vi "PCSLauncher.ProcPeriodic.vi"(0 "i ref in":refnum<vi>, 3 "ms timeout (100)":i32=100, 5 "error in (no error)":errorcluster) -> (14 "i ref out":refnum<vi>, 17 "timed out":bool, 19 "error out":errorcluster)   [LabVIEW 2014, in "PCSLauncher.lvlib"]
doc: "This method serves to periodically do things like reading values from the HW. Methods that should be executed periodically should be called from THIS methode. Add code here."
uses:
  PCSLauncher.lvlib
  CS_Core/CSObj/CSObj.lvlib
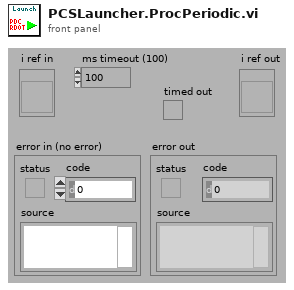
[diagram p1: front panel]
types:
  T1 = enum8{"Enabled", "Disabled", "Disabled and Grayed Out"}
  T2 = typedef "PCSLauncher.lvlib/PCSLauncher.i attribute.ctl" = cluster{"PCS Systems":cluster{"GUI Ref":refnum<vi>, "Super alive?":bool, "Start-GOG alive?":bool}[], "GUI Refs":cluster{"Delete":refnum<vi>, "Launch PCS":refnum<vi>}}
  T3 = cluster{"GUI Ref":refnum<vi>, "Super alive?":bool, "Start-GOG alive?":bool}[]
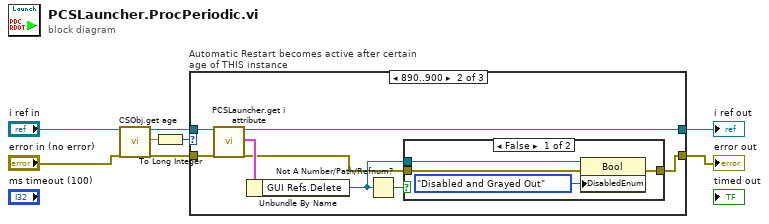
[diagram p0: block diagram]
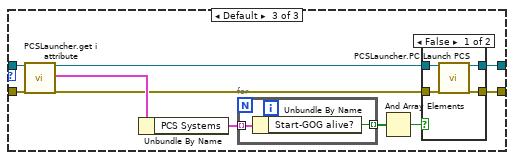
[diagram p4: hidden frame]
diagram:
  n1 = call "CSObj.get age.vi"("i ref in"="i ref in", "error in (no error)"="error in (no error)") -> ("i ref out"=w5:refnum<vi>, "age"=w1:dbl, "error out"=w3:errorcluster)  [unwired: 15 in]
  n2 = To Long Integer(number=w1) -> (32bit integer=w2:i32)
  n3 = case "Automatic Restart becomes active after certain age of THIS instance" shown="890..900" w2 {
    tunnel: [w10 w17 w30] -> w8
    tunnel: [w9 w11 w28] -> w7
    tunnel: w5 -> [w10 w18 w25]
    tunnel: w3 -> [w9 w16 w24]
    frame 0..889 {
    }
    frame 890..900 {
      n4 = call "PCSLauncher.get i attribute.vi"("i ref in"=w18, "error in (no error)"=w16) -> ("i ref out"=w17:refnum<vi>, "i attribute"=w15:T2, "error out"=w12:errorcluster)  [unwired: 15 in]
      n5 = Unbundle By Name(w15) -> ("GUI Refs.Delete"=w14:refnum<vi>)
      n6 = Not A Number/Path/Refnum?(number/path/refnum=w14) -> (NaN/Path/Refnum?=w13:bool)
      n7 = case shown="False" w13 {
        tunnel: w12 -> [w22 w23]
        tunnel: [w21 w23] -> w11
        tunnel: w14 -> [w20 _]
        frame False {
          n8 = property class="Bool"(reference=w20, error in=w22, "DisabledEnum"=T1."Disabled and Grayed Out" ("Disabled")) -> (error out=w21:errorcluster)  [unwired: 1 out]
        }
        frame True {
        }
      }
    }
    frame Default {
      n9 = call "PCSLauncher.get i attribute.vi"("i ref in"=w25, "error in (no error)"=w24) -> ("i ref out"=w31:refnum<vi>, "i attribute"=w33:T2, "error out"=w29:errorcluster)  [unwired: 15 in]
      n10 = Unbundle By Name(w33) -> ("PCS Systems"=w32:T3)
      n11 = for {
        tunnel: w32 -> [w41] mode=indexing
        tunnel: [w40] -> w27 mode=indexing
        n12 = Unbundle By Name(w41) -> ("Start-GOG alive?"=w40:bool)
      }
      n13 = And Array Elements(Boolean array=w27) -> (logical AND=w26:bool)
      n14 = case shown="False" w26 {
        tunnel: w31 -> [w37 w39]
        tunnel: [w36 w39] -> w30
        tunnel: w29 -> [w35 w38]
        tunnel: [w34 w38] -> w28
        frame False {
          n15 = call "PCSLauncher.PC Launch PCS.vi"("VI in"=w37, "error in (no error)"=w35) -> ("VI out"=w36:refnum<vi>, "error out"=w34:errorcluster)  [unwired: 16 in]
        }
        frame True {
        }
      }
    }
  }
  "error out" <- w7
  "i ref out" <- w8
